vi "CMN_BadParamMsg.vi"(5 "add list numbers":bool, 7 "valid params":string[](array[string]), 8 "error in (no error)":errorcluster, 10 "parameter":string) -> (0 "error out":errorcluster)   [LabVIEW 2016]
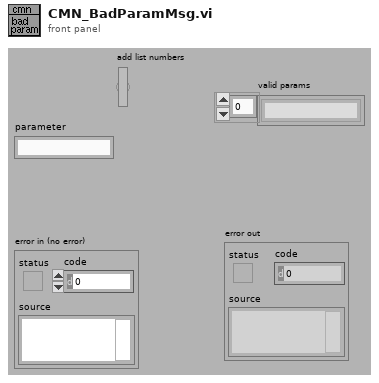
[diagram p1: front panel]
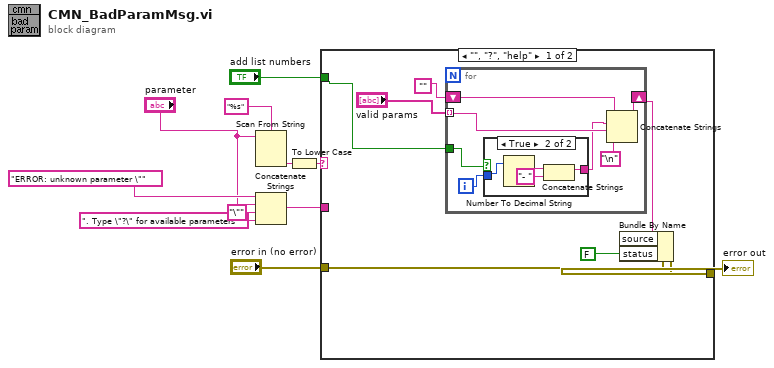
[diagram p0: block diagram]
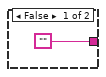
[diagram p2: hidden frame]
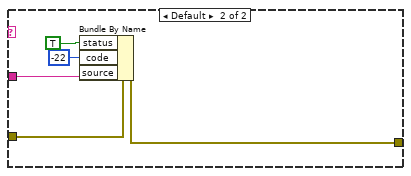
[diagram p3: hidden frame]
diagram:
  n1 = Scan From String(format string="%s", input string="parameter") -> (output 1=w4:string)  [unwired: 2 in, 4 out]
  n2 = Concatenate Strings("ERROR: unknown parameter \"" ("string"), "parameter", "\"" ("string"), ". Type \"?\" for available parameters" ("string")) -> (w7:string)
  n3 = To Lower Case(string=w4) -> (all lower case string=w3:string)
  n4 = case shown="\"\", \"?\", \"help\"" w3 {
    tunnel: "error in (no error)" -> [w18 w35]
    tunnel: [w17 w33] -> w10
    tunnel: w7 -> [_ w32]
    tunnel: "add list numbers" -> [w12 _]
    frame "", "?", "help" {
      n5 = for {
        tunnel: "valid params" -> [w25] mode=indexing
        shift-right: [w22] -> w14
        shift-left: "" -> [w24]
        tunnel: w12 -> [w21]
        i -> [w19]
        n6 = case shown="True" w21 {
          tunnel: ["" w27] -> w20
          tunnel: w19 -> [_ w30]
          frame False {
          }
          frame True {
            n7 = Number To Decimal String(number=w30) -> (decimal integer string=w29:string)  [unwired: 1 out]
            n8 = Concatenate Strings(w29, "- " ("string")) -> (w27:string)
          }
        }
        n9 = Concatenate Strings(w24, w20, w25, "\n") -> (w22:string)
      }
      n10 = Bundle By Name(cluster=w18, "source"=w14, "status"=FALSE) -> (w17:errorcluster)
    }
    frame Default {
      n11 = Bundle By Name(cluster=w35, "status"=TRUE, "code"=-22, "source"=w32) -> (w33:errorcluster)
    }
  }
  "error out" <- w10
